vi "Configure Comparator Swap.vi"(8 "error in (no error)":errorcluster, 10 "Comparator Swap State (F:Disable)":bool, 11 "VISA resource name":refnum<visa-resource-name>) -> (0 "error out":errorcluster, 3 "VISA resource name out":refnum<visa-resource-name>)   [LabVIEW 2017, in "Agilent E4980.lvlib"]
doc: "Exchanges the primary and secondary parameters of the measurement. \n\nFor example, if the measurement function is Cp-D when you use the parameter swap feature, the measurement function becomes D-Cp. After the swap, the comparator uses up to nine sets of limits for parameter D and one set of limit for parameter Cp."
uses:
  Agilent E4980.lvlib
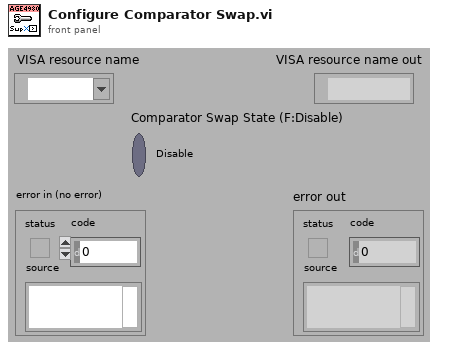
[diagram p1: front panel]
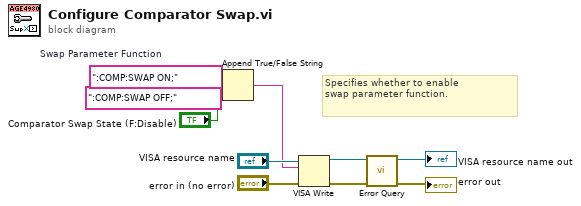
[diagram p0: block diagram]
diagram:
  w9 = ":COMP:SWAP ON;"  # Swap Parameter Function
  # "Specifies whether to enable\nswap parameter function."
  n1 = Append True/False String(1:"Comparator Swap State (F:Disable)", 2:":COMP:SWAP OFF;" ("true string"), 3:w9) -> (0:w1:string)  [unwired: 1 in]
  n2 = VISA Write(VISA resource name="VISA resource name", write buffer=w1, error in (no error)="error in (no error)") -> (VISA resource name out=w5:refnum<visa-resource-name>, error out=w4:errorcluster)  [unwired: 1 out]
  n3 = call "Error Query.vi"("error in (no error)"=w4, "VISA resource name"=w5) -> ("error out"=→"error out":errorcluster, "VISA resource name out"=→"VISA resource name out":refnum<visa-resource-name>)  [unwired: 6 in, 2 out]
